vi "FL_Decode_RAW_to_DEC_for_saving.vi"(0 "Sensor board size":string="Small", 1 "IO ports config":bool[](array[boolean]), 2 "Input timestamp":timestamp, 3 "Input string":string, 4 "Alternative magnets orientation and offset":bool, 5 "Error In":errorcluster) -> (6 "Output string leftover":string, 7 "DEC output cluster":T1, 8 "Error Out":errorcluster)   [LabVIEW 2016]
panel:
  out "TTL ins":bool[](array[boolean])
  out "TTL outs":bool[](array[boolean])
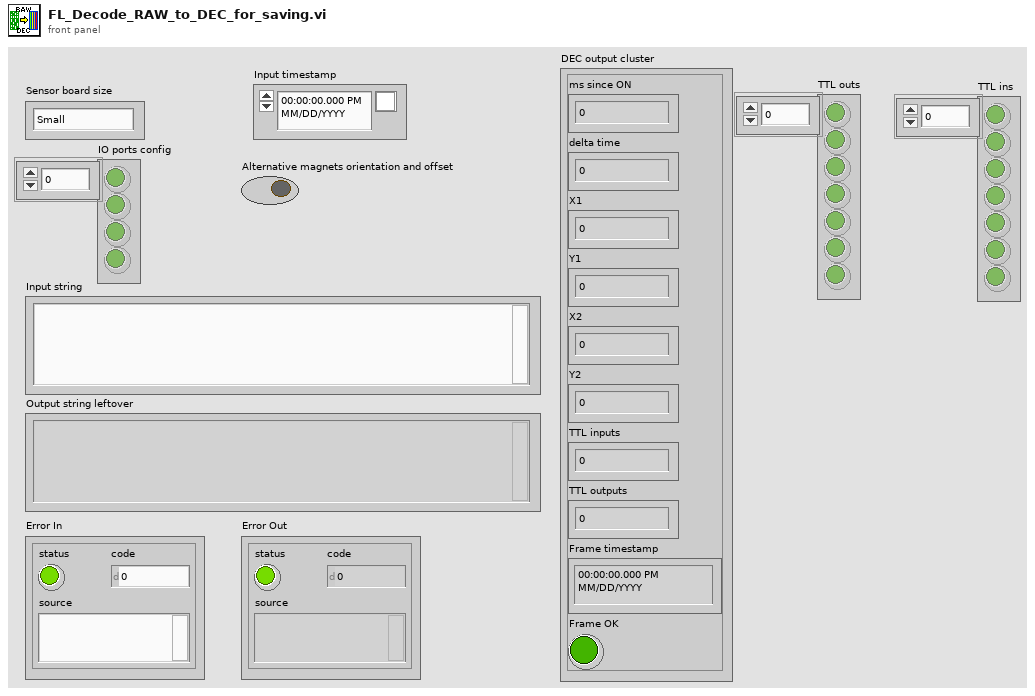
[diagram p1: front panel]
types:
  T1 = cluster{"ms since ON":u32, "delta time":u32, "X1":sgl, "Y1":sgl, "X2":sgl, "Y2":sgl, "TTL inputs":u8, "TTL outputs":u8, "Frame timestamp":timestamp, "Frame OK":bool}
  T2 = cluster{"ms since ON":u32, "delta time":u32, "X1":sgl, "Y1":sgl, "X2":sgl, "Y2":sgl, "TTL IO status":u8, "Frame timestamp":timestamp, "Frame OK":bool}
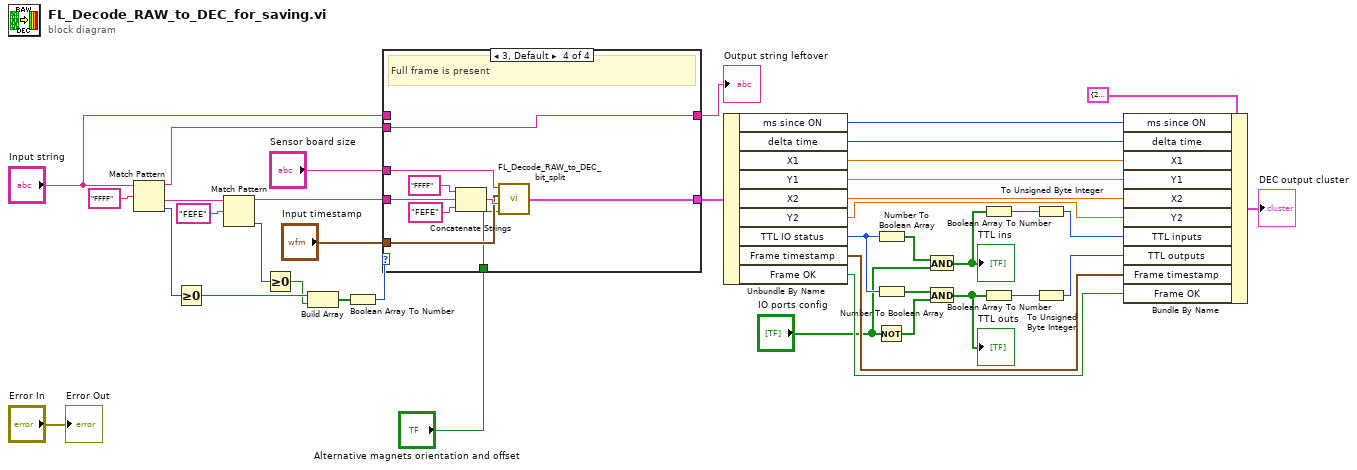
[diagram p0: block diagram]
diagram:
  n1 = Match Pattern(string="Input string", regular expression="FFFF") -> (before substring=w27:string, after substring=w28:string, offset past match=w32:i32)  [unwired: 1 in, 1 out]
  n2 = Greater Or Equal To 0?(x=w32) -> (x >= 0?=w37:bool)
  n3 = Match Pattern(string=w28, regular expression="FEFE") -> (before substring=w31:string, offset past match=w33:i32)  [unwired: 1 in, 2 out]
  n4 = Greater Or Equal To 0?(x=w33) -> (x >= 0?=w36:bool)
  n5 = Build Array(w37, w36) -> (w34:bool[])
  n6 = Boolean Array To Number(Boolean array=w34) -> (number=w35:u32)
  n7 = case shown="3, Default" w35 {
    tunnel: w31 -> [_ _ _ w50]
    tunnel: [_ _ _ w51] -> w23
    tunnel: "Input timestamp" -> [_ _ _ w45]
    tunnel: [w40 w41 w42 w46] -> w29
    tunnel: w27 -> [_ _ _ w46]
    tunnel: "Input string" -> [w40 w41 w42 _]
    tunnel: "Sensor board size" -> [_ _ _ w44]
    tunnel: "Alternative magnets orientation and offset" -> [_ _ _ w43]
    frame 0 {
      # "Neither beginning, nor ending of frame is present"
    }
    frame 1 {
      # "Only frame beginning is present"
    }
    frame 2 {
      # "Only frame end is present"
    }
    frame 3, Default {
      # "Full frame is present"
      n8 = Concatenate Strings("FFFF" ("string"), w50, "FEFE" ("string")) -> (w49:string)
      n9 = call "FL_Decode_RAW_to_DEC_bit_split.vi"("Alternative magnets orientation and offset"=w43, "Read buffer text to decode"=w49, "Input timestamp"=w45, "Sensor board size"=w44) -> ("DEC output cluster"=w51:T2)
    }
  }
  "Output string leftover" <- w29
  n10 = Unbundle By Name(w23) -> ("ms since ON"=w20:u32, "delta time"=w19:u32, "X1"=w18:sgl, "Y1"=w17:sgl, "X2"=w16:sgl, "Y2"=w15:sgl, "TTL IO status"=w11:u8, "Frame timestamp"=w14:timestamp, "Frame OK"=w13:bool)
  n11 = Not(x="IO ports config") -> (.not. x?=w8:bool[])
  n12 = Number To Boolean Array(number=w11) -> (Boolean array=w10:bool[])
  n13 = Number To Boolean Array(number=w11) -> (Boolean array=w12:bool[])
  n14 = And(x=w10, y="IO ports config") -> (x .and. y?=w5:bool[])
  "TTL ins" <- w5
  n15 = And(x=w12, y=w8) -> (x .and. y?=w7:bool[])
  "TTL outs" <- w7
  n16 = Boolean Array To Number(Boolean array=w5) -> (number=w4:u32)
  n17 = Boolean Array To Number(Boolean array=w7) -> (number=w6:u32)
  n18 = To Unsigned Byte Integer(number=w4) -> (unsigned 8bit integer=w3:u8)
  n19 = To Unsigned Byte Integer(number=w6) -> (unsigned 8bit integer=w2:u8)
  n20 = Bundle By Name(cluster=T1 {"ms since ON"=21424124, "delta time"=12, "X1"=-25.617287, "Y1"=-34.72222, "X2"=-30.650688, "Y2"=38.869858, "TTL inputs"=4, "TTL outputs"=0, "Frame timestamp"=timestamp(3611917532.9919057 s since 1904-01-01), "Frame OK"=TRUE} ("DEC output cluster"), "ms since ON"=w20, "delta time"=w19, "X1"=w18, "Y1"=w17, "X2"=w16, "Y2"=w15, "TTL inputs"=w3, "TTL outputs"=w2, "Frame timestamp"=w14, "Frame OK"=w13) -> (→"DEC output cluster":T1)
  "Error Out" <- "Error In"
